vi "Read Excel data.vi"(11 "file path (dialog if empty)":path) -> (0 "Number of rows":i32, 2 "Voltage Offsets":dbl[][](array[numeric]), 3 "Chirp Durations":dbl[][](array[numeric]), 5 "Multiplier":dbl[][](array[numeric]))   [LabVIEW 2017]
uses:
  <vilib>/Utility/file.llb/Read Delimited Spreadsheet (DBL).vi
panel:
  out "Plot Group":dbl[][](array[numeric])
  out "array w/o headers":dbl[][](array[numeric])
  out "all rows":dbl[][](array[numeric])
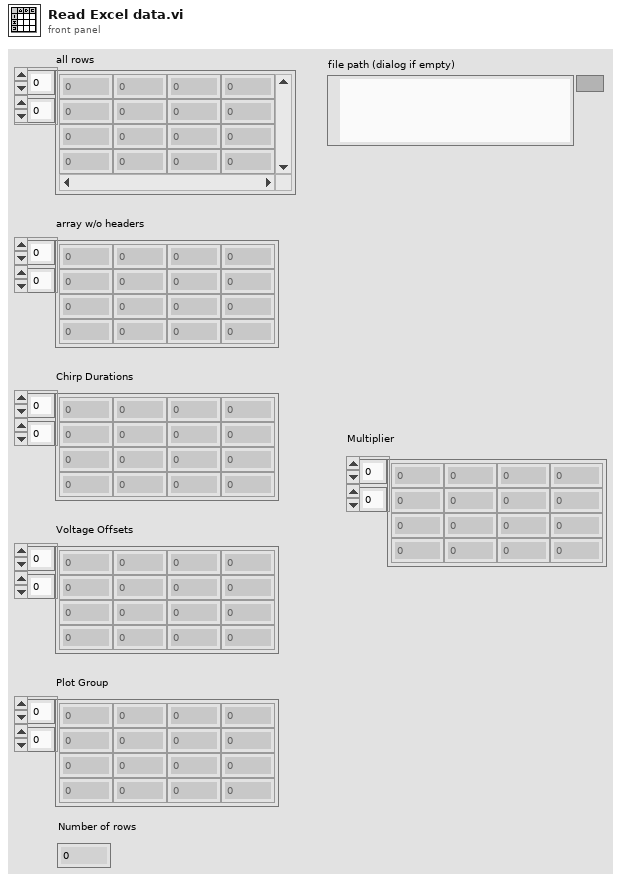
[diagram p1: front panel]
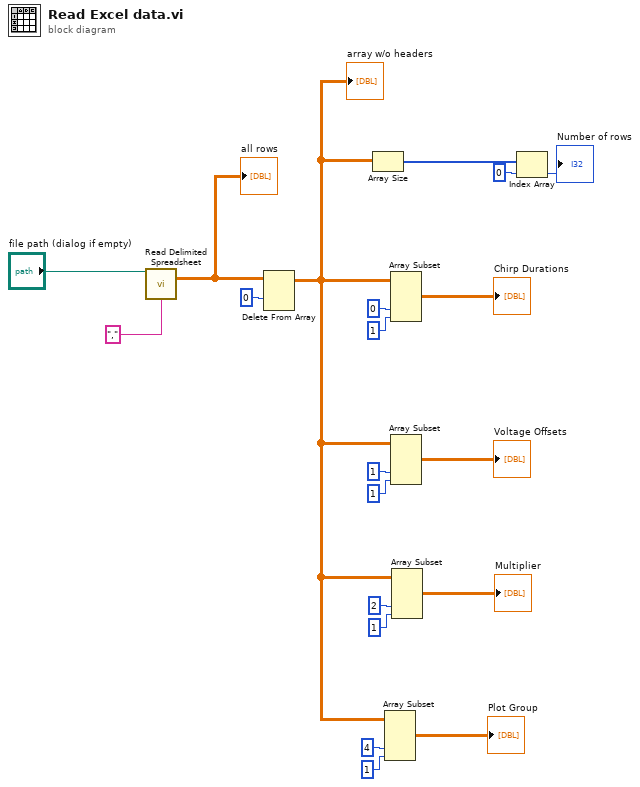
[diagram p0: block diagram]
diagram:
  n1 = call-poly <vilib>:"Read Delimited Spreadsheet.vi"("file path (dialog if empty)"="file path (dialog if empty)", "delimiter (\\t)"="," ("delimiter (\\t)")) -> ("all rows"=w20:dbl[][])  [unwired: 8 in, 5 out]
  "all rows" <- w20
  n2 = Delete From Array(array=w20, index (row)=0) -> (array with subset deleted=w1:dbl[][])  [unwired: 2 in, 1 out]
  "array w/o headers" <- w1
  n3 = Array Size(array=w1) -> (size(s)=w8:i32[])
  n4 = Array Subset(array=w1, index (col)=4 ("index"), length (col)=1 ("length")) -> (→"Plot Group":dbl[][])  [unwired: 2 in]
  n5 = Array Subset(array=w1, index (col)=0 ("index"), length (col)=1 ("length")) -> (→"Chirp Durations":dbl[][])  [unwired: 2 in]
  n6 = Array Subset(array=w1, index (col)=1 ("index"), length (col)=1 ("length")) -> (→"Voltage Offsets":dbl[][])  [unwired: 2 in]
  n7 = Array Subset(array=w1, index (col)=2 ("index"), length (col)=1 ("length")) -> (→"Multiplier":dbl[][])  [unwired: 2 in]
  n8 = Index Array(array=w8, index=0) -> (element=→"Number of rows":i32)
